vi "AddConnection.vi"(5 "data":T3={"New Subscriber"={"Caller ID"="", "Topic Name"="", "Protocol"="", "URIs"="", "ID"=refnum}, "ROS of Server"={"topic port"=0, "Node"="", "topic"="", "type"="", "node port"=0, "error "={"status"=FALSE, "code"=0, "source"=""}, "Direction"=enum."Node", "APIs"=[], "Update (ms)"=1, "write queue"=1}, "new port"=0}) -> (1 "Log":T2, 2 "MyState":T1)   [LabVIEW 2012]
uses:
  <userlib>/ROSforLV/ROS/Code/Console/Servers/ServerSubs/requestTopic.ctl
  <userlib>/ROSforLV/ROS/Code/SubVIs/_ROSControl.ctl
  <userlib>/ROSforLV/ROS/Code/SubVIs/_ROSDirection.ctl
  <userlib>/ROSforLV/ROS/Code/Console/Servers/ServerSubs/ROSLog.ctl
  <userlib>/ROSforLV/ROS/Code/Console/Servers/ServerSubs/MyState.ctl
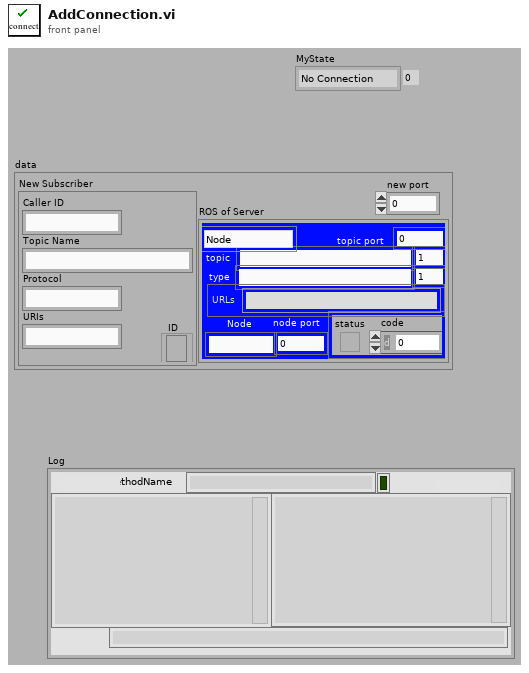
[diagram p1: front panel]
types:
  T1 = typedef "MyState.ctl" = enum16{"No Connection", "Registered", "Connected", "Close"}
  T2 = typedef "ROSLog.ctl" = cluster{"Sent":string, "Reply":string, "MethodName":string, "success":bool, "Dir1":string, "Dir2":string, "Time Stamp":string, "error":errorcluster, "Preamble":string}
  T3 = typedef "requestTopic.ctl" = cluster{"New Subscriber":cluster{"Caller ID":string, "Topic Name":string, "Protocol":string, "URIs":string, "ID":refnum<k5>}, "ROS of Server":T4, "new port":u16}
  T4 = typedef "_ROSControl.ctl" = cluster{"topic port":u16, "Node":string, "topic":string, "type":string, "node port":u32, "error ":errorcluster, "Direction":T5, "APIs":string[], "Update (ms)":u16, "write queue":u16}
  T5 = typedef "_ROSDirection.ctl" = enum16{"Node", "Publisher", "Subscriber", "Service Client"}
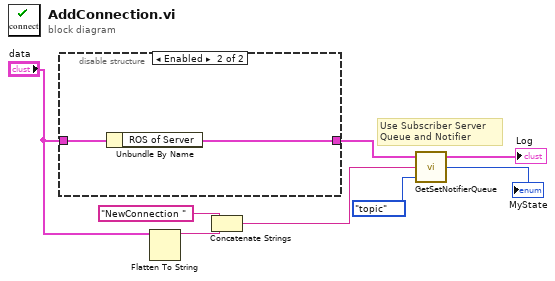
[diagram p0: block diagram]
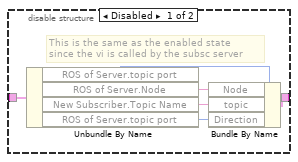
[diagram p2: hidden frame]
diagram:
  # "Use Subscriber Server \nQueue and Notifier"
  n1 = disable-structure shown="Enabled" {
    disable-tunnel: "data" -> [w11 w16]
    disable-tunnel: [w9 w15] -> w1
    frame Disabled {
      # "This is the same as the enabled state\nsince the vi is called by the subsc server"
      n2 = Unbundle By Name(w11) -> ("ROS of Server.topic port"=w10:u16, "ROS of Server.Node"=w12:string, "New Subscriber.Topic Name"=w14:string, "ROS of Server.topic port"=w13:u16)
      n3 = Bundle By Name(cluster=w10, "Node"=w12, "topic"=w14, "Direction"=w13) -> (w9:cluster{})
    }
    frame Enabled {
      n4 = Unbundle By Name(w16) -> ("ROS of Server"=w15:T4)
    }
  }
  n5 = Flatten To String(anything="data") -> (data string=w8:string)  [unwired: 3 in, 2 out]
  n6 = Concatenate Strings("NewConnection " ("element"), w8) -> (w5:string)
  n7 = call <userlib>:"GetSetNotifierQueue.vi"("Name"=enum16{"topic", "node"}."topic", "Command"=w5, "ROS"=w1) -> ("MyState"=→"MyState":T1, "Log"=→"Log":T2)  [unwired: 1 in]
